vi "configure.vi"(4 "error in (no error)":errorcluster, 5 "DPP Configuration":T1={"reset_recovery_time"=300, "edge_peaking_time"=1, "flat_top"=6, "peaking_time"=10, "gain"=1.0, "max_risetime"=30.0, "fast_filter_thr"=25, "zero_peak_freq"=0.0, "inverted_input"=0, "base_offset"=0, "reset_threshold"=0, "overflow_recovery"=30, "tail_coefficient"=0.0, "energy_filter_thr"=25, "energy_baseline_thr"=25, "max_peaking_time"=10, "edge_flat_top"=1, "time_constant"=0.0, "baseline_samples"=0, "other_param"=0}, 6 "Board":u16=25, 7 "identifier":string) -> (1 "function return":u32, 3 "error out":errorcluster)   [LabVIEW 2015, in "XGL_DPP.lvlib"]
doc: "EXTERN DECLSPEC uint32_t CALL_CONV configure(const char * identifier, uint16_t Board, const configuration cfg);"
uses:
  XGL_DPP.lvlib
  XGL_DPP.dll
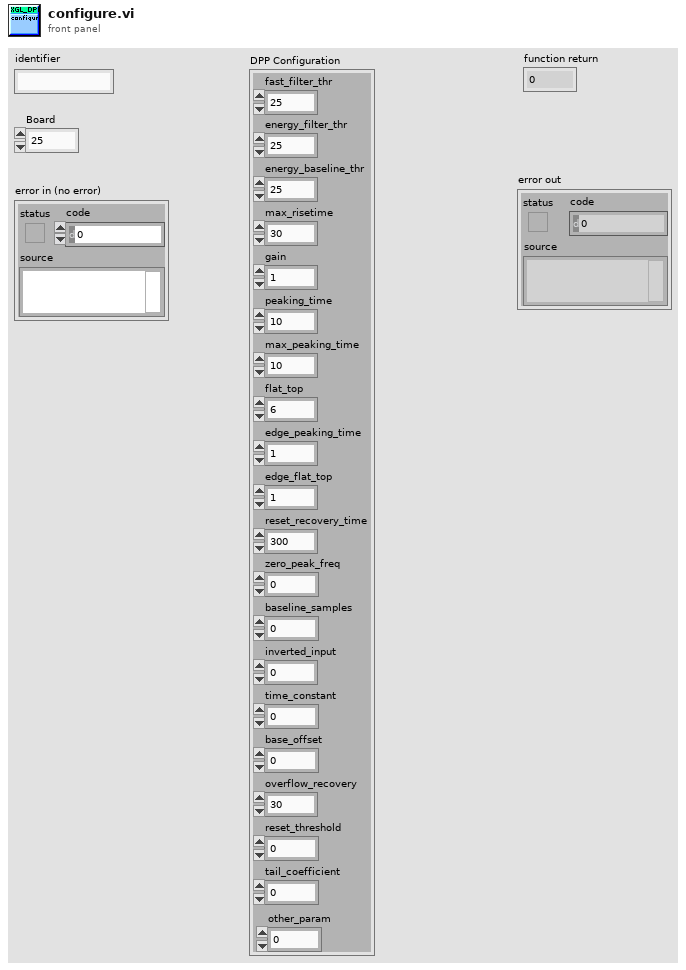
[diagram p1: front panel]
types:
  T1 = cluster{"reset_recovery_time":u32, "edge_peaking_time":u32, "flat_top":u32, "peaking_time":u32, "gain":dbl, "max_risetime":dbl, "fast_filter_thr":u32, "zero_peak_freq":dbl, "inverted_input":u8, "base_offset":u32, "reset_threshold":u32, "overflow_recovery":u32, "tail_coefficient":dbl, "energy_filter_thr":u32, "energy_baseline_thr":u32, "max_peaking_time":u32, "edge_flat_top":u32, "time_constant":dbl, "baseline_samples":u32, "other_param":u32}
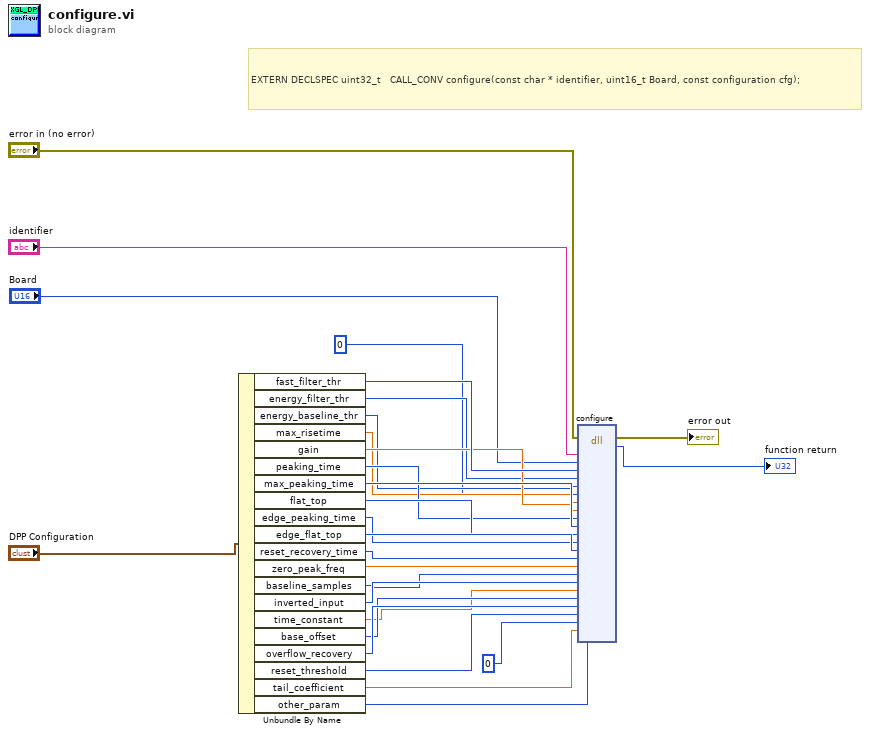
[diagram p0: block diagram]
diagram:
  # "EXTERN DECLSPEC uint32_t   CALL_CONV configure(const char * identifier, uint16_t Board, const configuration cfg);"
  n1 = Unbundle By Name("DPP Configuration") -> ("fast_filter_thr"=w23:u32, "energy_filter_thr"=w5:u32, "energy_baseline_thr"=w6:u32, "max_risetime"=w7:dbl, "gain"=w8:dbl, "peaking_time"=w9:u32, "max_peaking_time"=w10:u32, "flat_top"=w11:u32, "edge_peaking_time"=w12:u32, "edge_flat_top"=w13:u32, "reset_recovery_time"=w14:u32, "zero_peak_freq"=w15:dbl, "baseline_samples"=w16:u32, "inverted_input"=w17:u8, "time_constant"=w18:dbl, "base_offset"=w19:u32, "overflow_recovery"=w20:u32, "reset_threshold"=w21:u32, "tail_coefficient"=w22:dbl, "other_param"=w2:u32)
  n2 = dll-call lib="D:/Users/XRF/Desktop/Dante_acquire4/libs/Dante/XGL_DPP.*" fn="configure"(error in="error in (no error)", "identifier"="identifier", "Board"="Board", "fast_filter_thr"=w23, "energy_filter_thr"=w5, "energy_baseline_thr"=w6, "@dummy@"=i8 0 ("@dummy control@"), "max_risetime"=w7, "gain"=w8, "peaking_time"=w9, "max_peaking_time"=w10, "flat_top"=w11, "edge_peaking_time"=w12, "edge_flat_top"=w13, "reset_recovery_time"=w14, "zero_peak_freq"=w15, "baseline_samples"=w16, "inverted_input"=w17, "time_constant"=w18, "base_offset"=w19, "overflow_recovery"=w20, "reset_threshold"=w21, "@dummy@"=i8 0 ("@dummy control@"), "tail_coefficient"=w22, "other_param"=w2) -> (error out=→"error out":errorcluster, "return type"=→"function return":u32)  [unwired: 26 in, 1 out]
